vi "SNV_NA_2_0a.vi"(8 "ID In":string, 11 "Serial Port Select":refnum<visa-resource-name>) -> ()   [LabVIEW 2013]
uses:
  <vilib>/Utility/error.llb/DialogType.ctl
  instr.lib/lvserial/lvserial.lvlib
  <vilib>/Utility/miscctls.llb/LVPointDoubleTypeDef.ctl
panel:
  in  "stop":bool
  in  "External\nAtten.":dbl
  in  "Y Max":dbl=15.0
  in  "Y Min":dbl=-60.0
  in  "Auto\nY Axis":bool
  in  "File\nSave":bool
  in  "Take Cal\nData":bool
  in  "Cal On":bool
  in  "Trace\nHold":bool
  in  "#Points":dbl(ring)=100.0 items=["10"=10.0, "50"=50.0, "100"=100.0, "200"=200.0, "500"=500.0, "1000"=1000.0]
  in  "Stop":dbl=4000.0 min=34.0 max=4500.0
  in  "Start":dbl=50.0 min=34.0 max=4500.0
  out "ID":string
  in  "RF Power (dB)":dbl(slide)=-31.5 min=-31.5 max=0.0 step=0.5
  in  "Markers":bool=TRUE
  out "Delta":T1
  out "Cursor 2":T1
  out "Cursor 1":T1
  in  "RUN":bool=TRUE
  in  "comstop":bool
  out "CalData":cluster{dbl[], dbl[]}
  out "Trace":cluster{dbl[], dbl[]}
  out "scope":cluster{dbl[], "trace":dbl[]}[](graph)
  # "v2.0a"
  # "(MHz)"
  # "Windfreak"
  # "Min"
  # "Max"
  # "Technologies, LLC"
  # "2018"
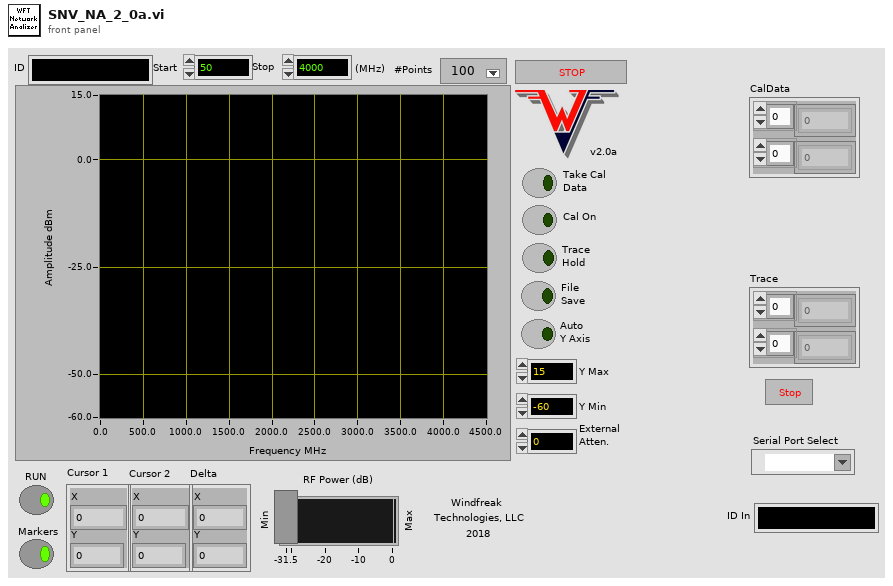
[diagram p1: front panel]
types:
  T1 = typedef "LVPointDoubleTypeDef.ctl" = cluster{"X":dbl, "Y":dbl}
  T2 = enum8{"Enabled", "Disabled", "Disabled and Grayed Out"}
  T3 = typedef "DialogType.ctl" = u16
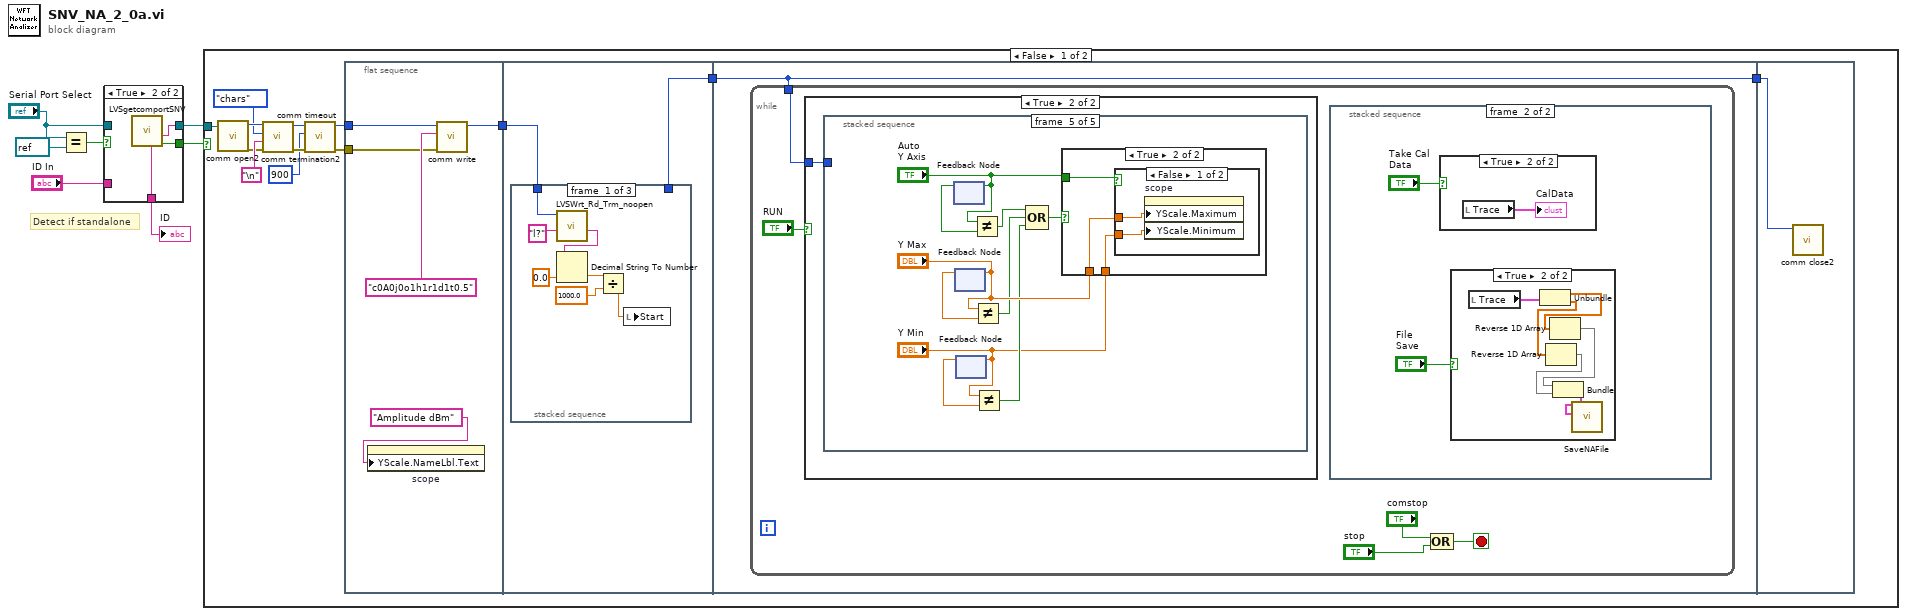
[diagram p0: block diagram]
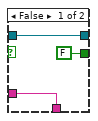
[diagram p2: hidden frame]
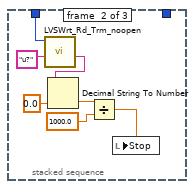
[diagram p3: hidden frame]
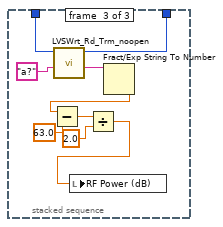
[diagram p4: hidden frame]
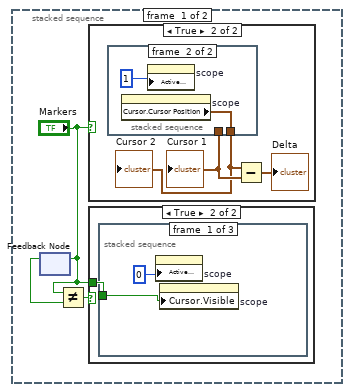
[diagram p5: hidden frame]
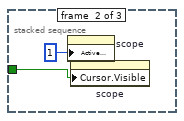
[diagram p7: hidden frame]
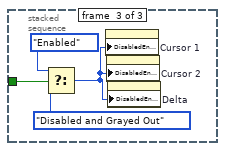
[diagram p8: hidden frame]
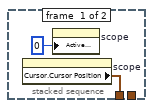
[diagram p10: hidden frame]
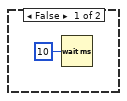
[diagram p13: hidden frame]
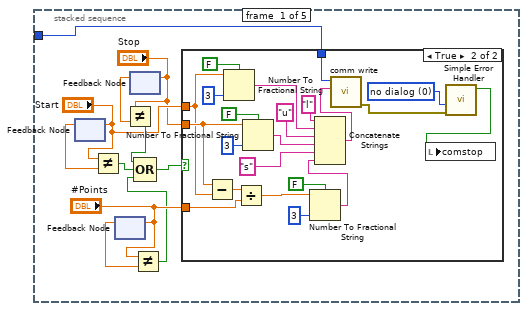
[diagram p14: hidden frame]
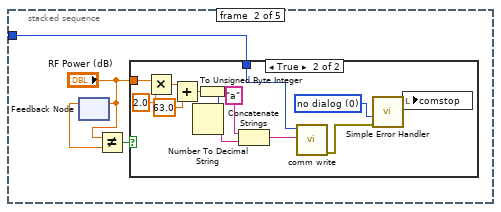
[diagram p16: hidden frame]
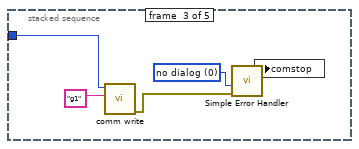
[diagram p18: hidden frame]
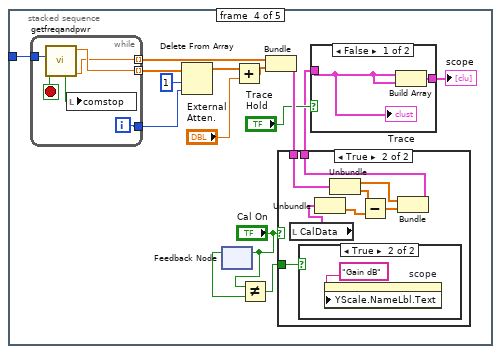
[diagram p19: hidden frame]
diagram:
  # "Detect if standalone"
  n1 = Equal?(x="Serial Port Select", y=refnum<visa-resource-name> refnum) -> (x = y?=w4:bool)
  n2 = case shown="True" w4 {
    tunnel: [w9 w13] -> w7
    tunnel: [FALSE ("No Devices") w12] -> w6
    tunnel: [w10 w11] -> w3
    tunnel: "ID In" -> [w10 _]
    tunnel: "Serial Port Select" -> [w9 _]
    frame False {
    }
    frame True {
      n3 = call "LVSgetcomportSNV.vi"() -> ("No Devices"=w12:bool, "Port"=w13:string, "Device"=w11:string)  [unwired: 9 in]
    }
  }
  "ID" <- w3
  n4 = case shown="False" w6 {
    tunnel: w7 -> [w20 _]
    frame False {
      n5 = call "comm open2.vi"("Comm Port Name"=w20) -> ("error out"=w21:errorcluster, "Comm Handle"=w22:u32)  [unwired: 4 in, 1 out]
      n6 = call "comm termination2.vi"("error in (no error)"=w21, "termination"="\n", "Termination Mode"=enum16{"none", "chars", "string", "regex"}."chars", "Comm Handle"=w22) -> ("error out"=w18:errorcluster, "dup Comm Handle"=w17:u32)  [unwired: 6 in]
      n7 = call "comm timeout.vi"("error in (no error)"=w18, "Timeout"=u32 900, "Comm Handle"=w17) -> ("error out"=w14:errorcluster, "dup Comm Handle"=w16:u32)  [unwired: 7 in]
      n8 = flat-sequence {
        tunnel: w16 -> [w30]
        tunnel: [w28] -> w24
        tunnel: w14 -> [w27]
        tunnel: [w32] -> w26
        tunnel: w24 -> [w33]
        tunnel: w26 -> [w57]
        tunnel: [w57] -> w25
        tunnel: w25 -> [w202]
        frame #0 {
          n9 = property on="scope" class="XYGraph (strict)"("YScale.NameLbl.Text"="Amplitude dBm" ("Y Scale.Name Label.Text")) -> ()  [unwired: 2 in, 2 out]
          n10 = call "comm write.vi"("error in (no error)"=w27, "string to write"="c0A0j0o1h1r1d1t0.5" ("string"), "Comm Handle"=w30) -> ("dup Comm Handle"=w28:u32)  [unwired: 6 in, 2 out]
        }
        frame #1 {
          n11 = stacked-sequence {
            tunnel: w33 -> [w35 w42 w50]
            tunnel: [_ _ w48] -> w32
            frame #0 {
              n12 = call "LVSWrt_Rd_Trm_noopen.vi"("WriteBuf"="l?" ("write buffer"), "Comm Handle"=w35) -> ("string read"=w34:string)  [unwired: 6 in, 2 out]
              n13 = Decimal String To Number(string=w34, default (0L)=0.0 ("default (0 I32)")) -> (number=w39:dbl)  [unwired: 1 in, 1 out]
              n14 = Divide(x=w39, y=1000.0) -> (x/y=w37:dbl)
              n15 = local write "Start"(w37) -> ()
            }
            frame #1 {
              n16 = call "LVSWrt_Rd_Trm_noopen.vi"("WriteBuf"="u?" ("write buffer"), "Comm Handle"=w42) -> ("string read"=w41:string)  [unwired: 6 in, 2 out]
              n17 = Decimal String To Number(string=w41, default (0L)=0.0 ("default (0 I32)")) -> (number=w46:dbl)  [unwired: 1 in, 1 out]
              n18 = Divide(x=w46, y=1000.0) -> (x/y=w44:dbl)
              n19 = local write "Stop"(w44) -> ()
            }
            frame #2 {
              n20 = call "LVSWrt_Rd_Trm_noopen.vi"("WriteBuf"="a?" ("write buffer"), "Comm Handle"=w50) -> ("string read"=w49:string, "Comm Handle Out"=w48:u32)  [unwired: 6 in, 1 out]
              n21 = Fract/Exp String To Number(string=w49) -> (number=w56:dbl)  [unwired: 3 in, 1 out]
              n22 = Subtract(x=w56, y=63.0) -> (x-y=w55:dbl)
              n23 = Divide(x=w55, y=2.0) -> (x/y=w52:dbl)
              n24 = local write "RF Power (dB)"(w52) -> ()
            }
          }
        }
        frame #2 {
          n25 = while {
            tunnel: w57 -> [w61]
            stop <- w58 stop-if-true
            n26 = case shown="True" "RUN" {
              tunnel: w61 -> [_ w92]
              frame False {
                n27 = Wait (ms)(milliseconds to wait=u32 10) -> ()  [unwired: 1 out]
              }
              frame True {
                n28 = stacked-sequence {
                  tunnel: w92 -> [w98 w126 w144 w160 _]
                  frame #0 {
                    n29 = feedback #1() -> (w103:dbl)  [unwired: 1 in]
                    n30 = feedback-in #1("Start") -> ()
                    n31 = Not Equal?(x="Start", y=w103) -> (x != y?=w102:bool)
                    n32 = feedback #2() -> (w95:dbl)  [unwired: 1 in]
                    n33 = feedback-in #2("#Points") -> ()
                    n34 = feedback #3() -> (w101:dbl)  [unwired: 1 in]
                    n35 = Not Equal?(x="Stop", y=w101) -> (x != y?=w100:bool)
                    n36 = feedback-in #3("Stop") -> ()
                    n37 = Not Equal?(x="#Points", y=w95) -> (x != y?=w93:bool)
                    n38 = Compound Arithmetic op=OR(w100, w102, w93) -> (w99:bool)
                    n39 = case shown="True" w99 {
                      tunnel: w98 -> [_ w106]
                      tunnel: "Start" -> [_ w117]
                      tunnel: "Stop" -> [_ w118]
                      tunnel: "#Points" -> [_ w110]
                      frame False {
                      }
                      frame True {
                        w109 = T3 0 items=["no dialog", "OK message", "continue or stop message", "OK message + warnings", "continue/stop + warnings"] ("type of dialog (OK msg:1)")
                        n40 = Subtract(x=w118, y=w117) -> (x-y=w116:dbl)
                        n41 = Number To Fractional String(use system decimal point (T)=FALSE, number=w117, precision (6)=i16 3) -> (F-format string=w123:string)  [unwired: 1 in]
                        n42 = Divide(x=w116, y=w110) -> (x/y=w112:dbl)
                        n43 = Number To Fractional String(use system decimal point (T)=FALSE, number=w118, precision (6)=i16 3) -> (F-format string=w119:string)  [unwired: 1 in]
                        n44 = Number To Fractional String(use system decimal point (T)=FALSE, number=w112, precision (6)=i16 3) -> (F-format string=w111:string)  [unwired: 1 in]
                        n45 = Concatenate Strings("l" ("string"), w123, "u" ("string"), w119, "s" ("string"), w111) -> (w104:string)
                        n46 = call "comm write.vi"("string to write"=w104, "Comm Handle"=w106) -> ("error out"=w105:errorcluster)  [unwired: 7 in, 2 out]
                        n47 = call <vilib>:"Simple Error Handler.vi"("type of dialog (OK msg:1)"=w109, "error in (no error)"=w105) -> ("error?"=w108:bool)  [unwired: 7 out]
                        n48 = local write "comstop"(w108) -> ()
                      }
                    }
                  }
                  frame #1 {
                    n49 = feedback #4() -> (w127:dbl)  [unwired: 1 in]
                    n50 = feedback-in #4("RF Power (dB)") -> ()
                    n51 = Not Equal?(x="RF Power (dB)", y=w127) -> (x != y?=w129:bool)
                    n52 = case shown="True" w129 {
                      tunnel: "RF Power (dB)" -> [_ w138]
                      tunnel: w126 -> [_ w131]
                      frame False {
                      }
                      frame True {
                        w133 = T3 0 items=["no dialog", "OK message", "continue or stop message", "OK message + warnings", "continue/stop + warnings"] ("type of dialog (OK msg:1)")
                        n53 = Multiply(x=w138, y=2.0) -> (x*y=w140:dbl)
                        n54 = Add(x=w140, y=63.0) -> (x+y=w142:dbl)
                        n55 = To Unsigned Byte Integer(number=w142) -> (unsigned 8bit integer=w135:u8)
                        n56 = Number To Decimal String(number=w135) -> (decimal integer string=w137:string)  [unwired: 1 in]
                        n57 = Concatenate Strings("a" ("element"), w137) -> (w132:string)
                        n58 = call "comm write.vi"("string to write"=w132, "Comm Handle"=w131) -> ("error out"=w130:errorcluster)  [unwired: 7 in, 2 out]
                        n59 = call <vilib>:"Simple Error Handler.vi"("type of dialog (OK msg:1)"=w133, "error in (no error)"=w130) -> ("error?"=w134:bool)  [unwired: 7 out]
                        n60 = local write "comstop"(w134) -> ()
                      }
                    }
                  }
                  frame #2 {
                    w147 = T3 0 items=["no dialog", "OK message", "continue or stop message", "OK message + warnings", "continue/stop + warnings"] ("type of dialog (OK msg:1)")
                    n61 = call "comm write.vi"("string to write"="g1" ("string"), "Comm Handle"=w144) -> ("error out"=w143:errorcluster)  [unwired: 7 in, 2 out]
                    n62 = call <vilib>:"Simple Error Handler.vi"("type of dialog (OK msg:1)"=w147, "error in (no error)"=w143) -> ("error?"=w146:bool)  [unwired: 7 out]
                    n63 = local write "comstop"(w146) -> ()
                  }
                  frame #3 {
                    n64 = while {
                      tunnel: w160 -> [w180]
                      tunnel: [w184] -> w162 mode=indexing
                      tunnel: [w183] -> w157
                      tunnel: [w182] -> w158 mode=indexing
                      i -> [w183]
                      stop <- w185 stop-if-true
                      n65 = call "getfreqandpwr.vi"("Comm Handle"=w180) -> ("Freq"=w182:dbl, "RF Detector Pwr dBm"=w184:dbl, "error?"=w181:bool, "EOS"=w185:bool)  [unwired: 7 in]
                      n66 = local write "comstop"(w181) -> ()
                    }
                    n67 = Delete From Array(array=w162, length=1, index=w157) -> (array with subset deleted=w153:dbl[])  [unwired: 1 out]
                    n68 = feedback #5() -> (w151:bool)  [unwired: 1 in]
                    n69 = feedback-in #5("Cal On") -> ()
                    n70 = Add(x=w153, y="External\nAtten.") -> (x+y=w154:dbl[])
                    n71 = Not Equal?(x="Cal On", y=w151) -> (x != y?=w149:bool)
                    n72 = Bundle(w158, w154) -> (w155:cluster{dbl[], dbl[]})  [unwired: 1 in]
                    n73 = case shown="True" "Cal On" {
                      tunnel: w155 -> [w164 w173]
                      tunnel: [w164 w168] -> w148
                      tunnel: w149 -> [w163 w166]
                      frame False {
                        n74 = case shown="False" w163 {
                          frame False {
                          }
                          frame True {
                            n75 = property on="scope" class="XYGraph (strict)"("YScale.NameLbl.Text"="Amplitude dBm" ("Y Scale.Name Label.Text")) -> ()  [unwired: 2 in, 2 out]
                          }
                        }
                      }
                      frame True {
                        n76 = local read "CalData"() -> (w167:cluster{dbl[], dbl[]})
                        n77 = case shown="True" w166 {
                          frame False {
                          }
                          frame True {
                            n78 = property on="scope" class="XYGraph (strict)"("YScale.NameLbl.Text"="Gain dB" ("Y Scale.Name Label.Text")) -> ()  [unwired: 2 in, 2 out]
                          }
                        }
                        n79 = Unbundle(w167) -> (w172:dbl[])  [unwired: 1 out]
                        n80 = Unbundle(w173) -> (w169:dbl[], w171:dbl[])
                        n81 = Subtract(x=w171, y=w172) -> (x-y=w170:dbl[])
                        n82 = Bundle(w169, w170) -> (w168:cluster{dbl[], dbl[]})  [unwired: 1 in]
                      }
                    }
                    n83 = case shown="False" "Trace\nHold" {
                      tunnel: [w176 w179] -> w159
                      tunnel: w148 -> [w175 w178]
                      frame False {
                        n84 = Build Array(w175, w175) -> (w176:cluster{dbl[], dbl[]}[])
                        "Trace" <- w175
                      }
                      frame True {
                        n85 = local read "Trace"() -> (w177:cluster{dbl[], dbl[]})
                        n86 = Build Array(w178, w177) -> (w179:cluster{dbl[], dbl[]}[])
                      }
                    }
                    "scope" <- w159
                  }
                  frame #4 {
                    n87 = feedback #6() -> (w186:bool)  [unwired: 1 in]
                    n88 = feedback-in #6("Auto\nY Axis") -> ()
                    n89 = feedback #7() -> (w188:dbl)  [unwired: 1 in]
                    n90 = feedback-in #7("Y Max") -> ()
                    n91 = feedback #8() -> (w189:dbl)  [unwired: 1 in]
                    n92 = feedback-in #8("Y Min") -> ()
                    n93 = Not Equal?(x="Auto\nY Axis", y=w186) -> (x != y?=w194:bool)
                    n94 = Not Equal?(x="Y Max", y=w188) -> (x != y?=w192:bool)
                    n95 = Not Equal?(x="Y Min", y=w189) -> (x != y?=w193:bool)
                    n96 = Compound Arithmetic op=OR(w194, w192, w193) -> (w191:bool)
                    n97 = case shown="True" w191 {
                      tunnel: "Auto\nY Axis" -> [_ w198]
                      tunnel: "Y Max" -> [_ w197]
                      tunnel: "Y Min" -> [_ w196]
                      frame False {
                      }
                      frame True {
                        n98 = case shown="False" w198 {
                          tunnel: w197 -> [w200 _]
                          tunnel: w196 -> [w199 _]
                          frame False {
                            n99 = property on="scope" class="XYGraph (strict)"("YScale.Maximum"=w200, "YScale.Minimum"=w199) -> ()  [unwired: 2 in, 2 out]
                          }
                          frame True {
                            n100 = property on="scope" class="XYGraph (strict)"("YScale.ScaleFit"=u8 1 ("Y Scale.Scale Fit")) -> ()  [unwired: 2 in, 2 out]
                          }
                        }
                      }
                    }
                  }
                }
              }
            }
            n101 = stacked-sequence {
              frame #0 {
                n102 = feedback #9() -> (w65:bool)  [unwired: 1 in]
                n103 = feedback-in #9("Markers") -> ()
                n104 = Not Equal?(x="Markers", y=w65) -> (x != y?=w64:bool)
                n105 = case shown="True" "Markers" {
                  frame False {
                  }
                  frame True {
                    n106 = stacked-sequence {
                      tunnel: [w78 _] -> w76
                      tunnel: [_ w80] -> w75
                      frame #0 {
                        n107 = property on="scope" class="XYGraph (strict)"() -> ("Cursor.Cursor Position"=w78:T1)  [unwired: 2 in, 2 out]
                        n108 = property on="scope" class="XYGraph (strict)"("Active Cursor"=u32 0) -> ()  [unwired: 2 in, 2 out]
                      }
                      frame #1 {
                        n109 = property on="scope" class="XYGraph (strict)"() -> ("Cursor.Cursor Position"=w80:T1)  [unwired: 2 in, 2 out]
                        n110 = property on="scope" class="XYGraph (strict)"("Active Cursor"=u32 1) -> ()  [unwired: 2 in, 2 out]
                      }
                    }
                    "Cursor 1" <- w76
                    "Cursor 2" <- w75
                    n111 = Subtract(x=w75, y=w76) -> (x-y=→"Delta":T1)
                  }
                }
                n112 = case shown="True" w64 {
                  tunnel: "Markers" -> [_ w66]
                  frame False {
                  }
                  frame True {
                    n113 = stacked-sequence {
                      tunnel: w66 -> [w68 w69 w74]
                      frame #0 {
                        n114 = property on="scope" class="XYGraph (strict)"("Active Cursor"=u32 0) -> ()  [unwired: 2 in, 2 out]
                        n115 = property on="scope" class="XYGraph (strict)"("Cursor.Visible"=w68) -> ()  [unwired: 2 in, 2 out]
                      }
                      frame #1 {
                        n116 = property on="scope" class="XYGraph (strict)"("Active Cursor"=u32 1) -> ()  [unwired: 2 in, 2 out]
                        n117 = property on="scope" class="XYGraph (strict)"("Cursor.Visible"=w69) -> ()  [unwired: 2 in, 2 out]
                      }
                      frame #2 {
                        n118 = Select(t=T2."Enabled" ("Disabled"), s=w74, f=T2."Disabled and Grayed Out" ("Disabled")) -> (s? t:f=w71:T2)
                        n119 = property on="Cursor 1" class="Clust (strict)"("DisabledEnum"=w71) -> ()  [unwired: 2 in, 2 out]
                        n120 = property on="Cursor 2" class="Clust (strict)"("DisabledEnum"=w71) -> ()  [unwired: 2 in, 2 out]
                        n121 = property on="Delta" class="Clust (strict)"("DisabledEnum"=w71) -> ()  [unwired: 2 in, 2 out]
                      }
                    }
                  }
                }
              }
              frame #1 {
                n122 = case shown="True" "Take Cal\nData" {
                  frame False {
                  }
                  frame True {
                    n123 = local read "Trace"() -> (→"CalData":cluster{dbl[], dbl[]})
                  }
                }
                n124 = case shown="True" "File\nSave" {
                  frame False {
                  }
                  frame True {
                    n125 = local read "Trace"() -> (w84:cluster{dbl[], dbl[]})
                    n126 = Unbundle(w84) -> (w89:dbl[], w88:dbl[])
                    n127 = Reverse 1D Array(array=w88) -> (reversed array=w86:dbl[])
                    n128 = Reverse 1D Array(array=w89) -> (reversed array=w87:dbl[])
                    n129 = Bundle(w87, w86) -> (w85:cluster{dbl[], dbl[]})  [unwired: 1 in]
                    n130 = call "SaveNAFile.vi"("XY"=w85) -> ()  [unwired: 7 in, 1 out]
                  }
                }
              }
            }
            n131 = Compound Arithmetic op=OR("comstop", "stop") -> (w58:bool)
          }
        }
        frame #3 {
          n132 = call "comm close2.vi"("Comm Handle"=w202) -> ()  [unwired: 6 in, 1 out]
        }
      }
    }
    frame True {
      n133 = Open VI Reference(vi path=path "NAfull.vi") -> (vi reference=w203:refnum<vi>)  [unwired: 5 in, 1 out]
      n134 = invoke class="VI" method="FP.Close"(reference=w203) -> ()  [unwired: 2 in, 3 out]
    }
  }
